vi "Add.vi"() -> ()   [LabVIEW 2019, in "MicronTemplateCore.lvclass"]
doc: "This is the VI description for the Add command, which can be queried by a client with\nCommand : Help, Payload: Add."
uses:
  MicronTemplateCore.lvclass
panel:
  out "Numeric3":dbl
  in  "Numeric2":dbl
  in  "Numeric1":dbl
  # "Add Two Numbers"
  # "This is a sample method to demonstrate querying and invocation of the command 'Add' from an external client (LabVIEW, Python or any other language). \n\nWhen the method is invoked, the front panel of the method would be shown in the UI of the service & would remain visible till the next command is invoked. This is done without any static linkage in the service. \n\nWhen you add a new method to the Core class, it would be immediately available for usage by the client without any additional configuration. \n\nGo ahead and try creating a subtract method in Core and try calling it from client!"
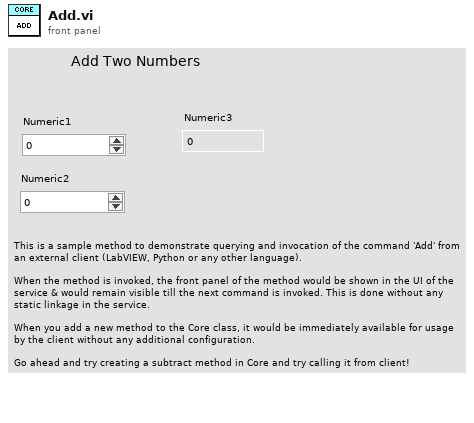
[diagram p1: front panel]
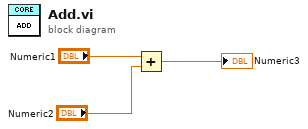
[diagram p0: block diagram]
diagram:
  n1 = Add(x="Numeric1", y="Numeric2") -> (x+y=→"Numeric3":dbl)
